vi "Ke2400 Voltage Current Setting.vi"(8 "error in (no error)":errorcluster, 9 "Current(mA)":dbl=60.0, 10 "Voltage(V)":dbl, 11 "VISA resource name":refnum<visa-resource-name>) -> (0 "error out":errorcluster, 3 "VISA resource name out":refnum<visa-resource-name>)   [LabVIEW 2012]
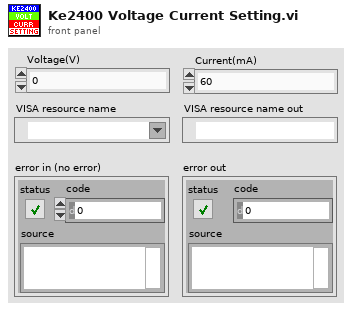
[diagram p1: front panel]
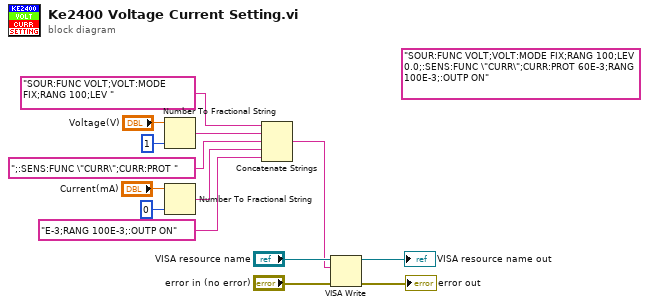
[diagram p0: block diagram]
diagram:
  (unwired) "SOUR:FUNC VOLT;VOLT:MODE FIX;RANG 100;LEV 0.0;:SENS:FUNC \"CURR\";CURR:PROT 60E-3;RANG 100E-3;:OUTP ON" ("write buffer")
  n1 = Number To Fractional String(number="Voltage(V)", precision (6)=i16 1) -> (F-format string=w6:string)  [unwired: 2 in]
  n2 = Number To Fractional String(number="Current(mA)", precision (6)=i16 0) -> (F-format string=w3:string)  [unwired: 2 in]
  n3 = Concatenate Strings("SOUR:FUNC VOLT;VOLT:MODE FIX;RANG 100;LEV " ("write buffer"), w6, ";:SENS:FUNC \"CURR\";CURR:PROT " ("write buffer"), w3, "E-3;RANG 100E-3;:OUTP ON" ("write buffer")) -> (w1:string)
  n4 = VISA Write(VISA resource name="VISA resource name", write buffer=w1, error in (no error)="error in (no error)") -> (VISA resource name out=→"VISA resource name out":refnum<visa-resource-name>, error out=→"error out":errorcluster)  [unwired: 1 out]
